vi "Send UNREGISTER.vi"(8 "error in (no error)":errorcluster, 9 "Unregister Request":T1, 10 "Message loop data (in)":T2, 11 "WAMP Client in":refnum<class "WAMP Client.lvclass">) -> (0 "error out":errorcluster, 2 "Message loop data (out)":T2, 3 "WAMP Client out":refnum<class "WAMP Client.lvclass">)   [LabVIEW 2021, in "wamplv.lvlib" / "WAMP Client.lvclass"]
uses:
  WAMP Client.lvclass
  TypeDef/Message Loop Shift Reg Data.ctl
  TypeDef/REGISTER Request Data.ctl
  API/TypeDefs/INVOCATION payload.ctl
  TypeDef/Success or error.ctl
  API/TypeDefs/Combined error.ctl
  API/TypeDefs/WAMP error.ctl
  TypeDef/Publish Requests Map.ctl
  TypeDef/PUBLISH Request Data.ctl
  TypeDef/PUBLISH result.ctl
  TypeDef/Endpoint Data.ctl
  TypeDef/CALL Request Map.ctl
  TypeDef/CALL Request Data.ctl
  API/TypeDefs/RESULT payload.ctl
  TypeDef/SUBSCRIBE Requests Map.ctl
  TypeDef/SUBSCRIBE Request Data.ctl
  TypeDef/Subscribe Result.ctl
  TypeDef/EVENT payload.ctl
  TypeDef/Subscriptions Map.ctl
  TypeDef/Subscription Details.ctl
  TypeDef/Unsubscribe Requests Map.ctl
  TypeDef/UNSUBSCRIBE Request Data.ctl
  TypeDef/UNSUBSCRIBE Result.ctl
  TypeDef/Unregister requests map.ctl
  TypeDef/Unregister request.ctl
  TypeDef/WAMP Message Codes.ctl
  WAMP Client.lvclass/WAMP Client.ctl
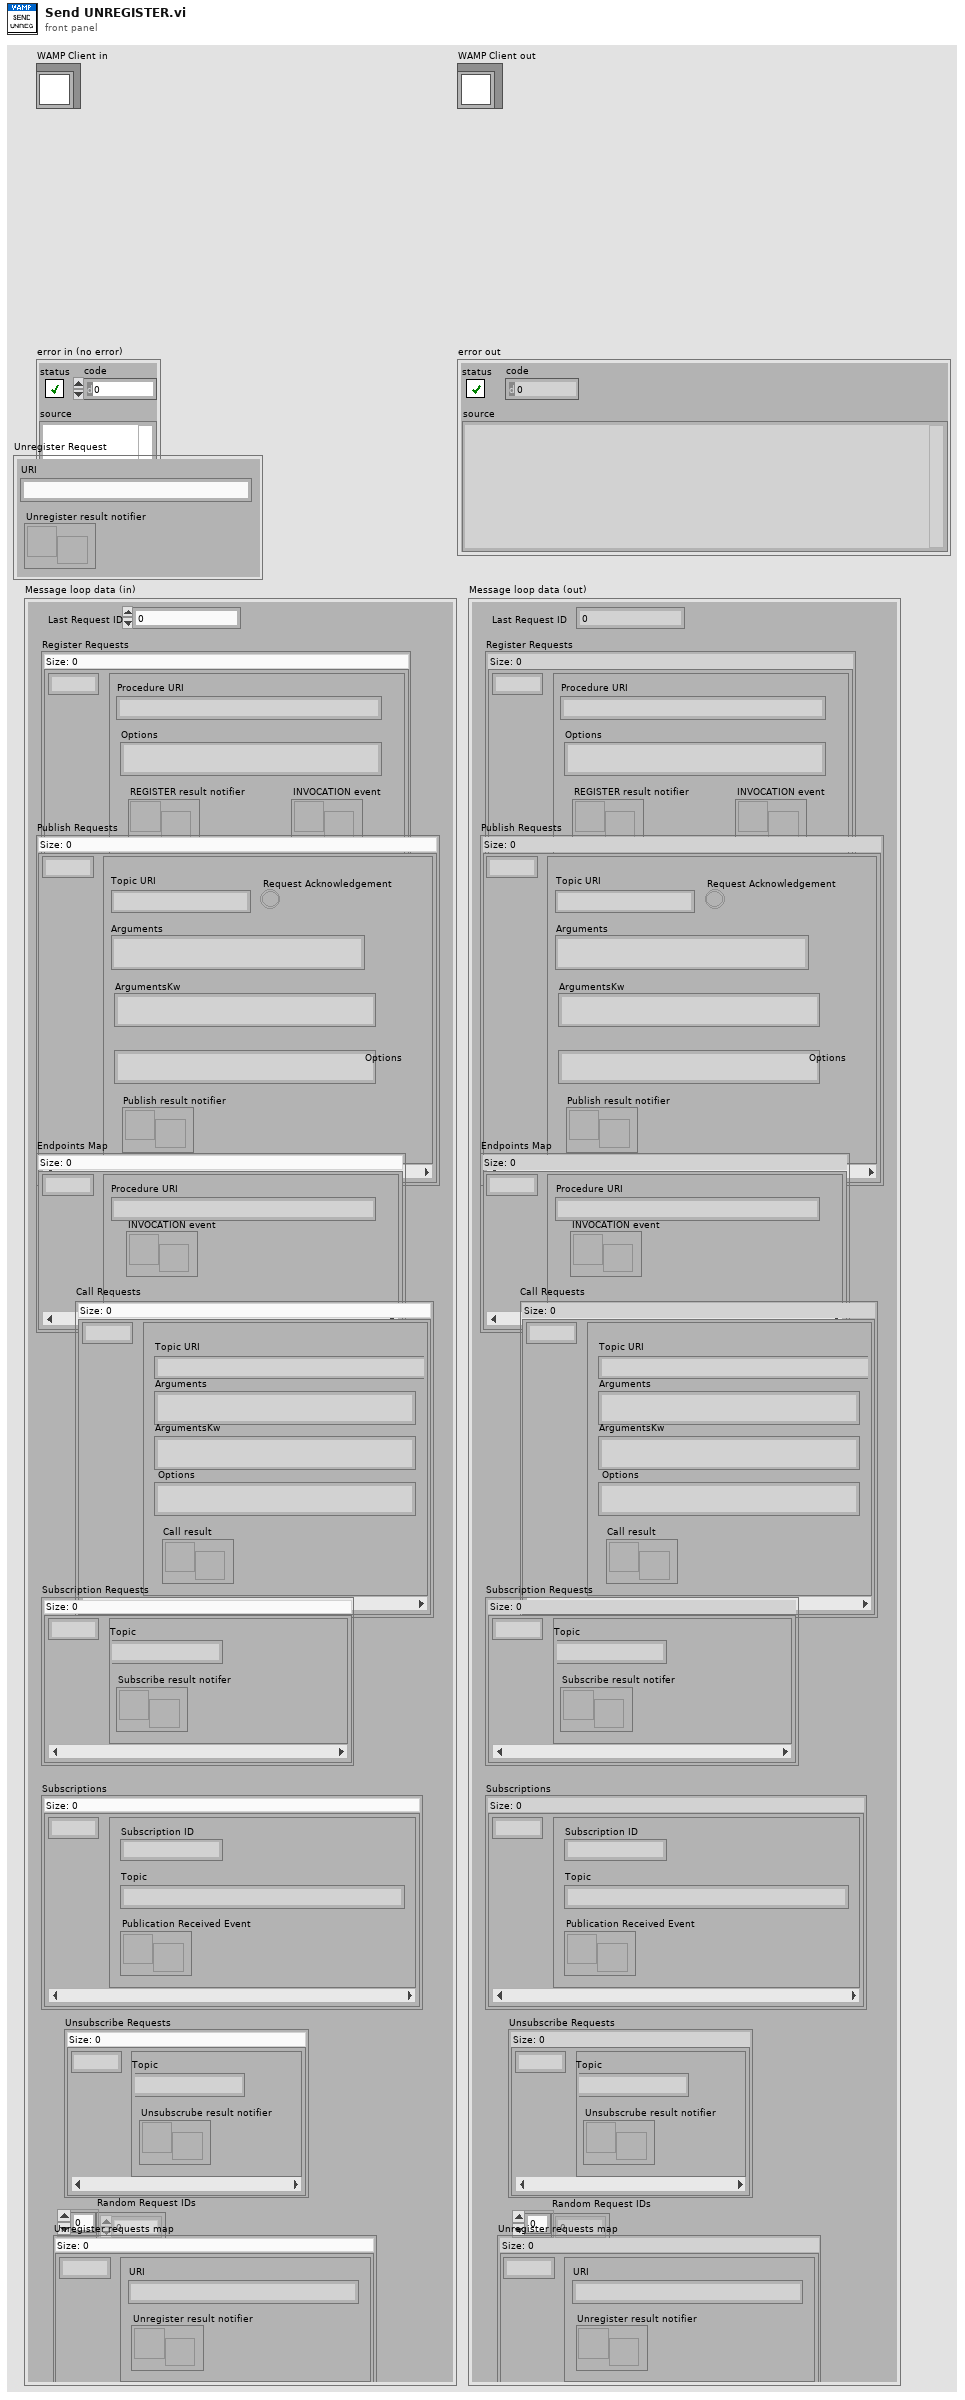
[diagram p1: front panel]
types:
  T1 = typedef "wamplv.lvlib/WAMP Client.lvclass/Unregister request.ctl" = cluster{"URI":string, "Unregister result notifier":refnum<notifier>}
  T2 = typedef "wamplv.lvlib/WAMP Client.lvclass/Message Loop Shift Reg Data.ctl" = cluster{"Last Request ID":u64, "Register Requests":map{u64, T3}, "Publish Requests":T4, "Endpoints Map":map{u64, T6}, "Call Requests":T7, "Subscription Requests":T9, "Subscriptions":T11, "Unsubscribe Requests":T13, "Random Request IDs":u64[], "Unregister requests map":T15}
  T3 = typedef "wamplv.lvlib/WAMP Client.lvclass/REGISTER Request Data.ctl" = cluster{"Procedure URI":string, "Options":string, "INVOCATION event":refnum<user-event>, "REGISTER result notifier":refnum<notifier>}
  T4 = typedef "wamplv.lvlib/WAMP Client.lvclass/Publish Requests Map.ctl" = map{u64, T5}
  T5 = typedef "wamplv.lvlib/WAMP Client.lvclass/PUBLISH Request Data.ctl" = cluster{"Topic URI":string, "Arguments":string, "ArgumentsKw":string, "Request Acknowledgement":bool, "Options":string, "Publish result notifier":refnum<notifier>}
  T6 = typedef "wamplv.lvlib/WAMP Client.lvclass/Endpoint Data.ctl" = cluster{"Procedure URI":string, "INVOCATION event":refnum<user-event>}
  T7 = typedef "wamplv.lvlib/WAMP Client.lvclass/CALL Request Map.ctl" = map{u64, T8}
  T8 = typedef "wamplv.lvlib/WAMP Client.lvclass/CALL Request Data.ctl" = cluster{"Topic URI":string, "Arguments":string, "ArgumentsKw":string, "Options":string, "Call result":refnum<notifier>}
  T9 = typedef "wamplv.lvlib/WAMP Client.lvclass/SUBSCRIBE Requests Map.ctl" = map{u64, T10}
  T10 = typedef "wamplv.lvlib/WAMP Client.lvclass/SUBSCRIBE Request Data.ctl" = cluster{"Topic":string, "Subscribe result notifer":refnum<notifier>}
  T11 = typedef "wamplv.lvlib/WAMP Client.lvclass/Subscriptions Map.ctl" = map{u64, T12}
  T12 = typedef "wamplv.lvlib/WAMP Client.lvclass/Subscription Details.ctl" = cluster{"Subscription ID":u64, "Topic":string, "Publication Received Event":refnum<user-event>}
  T13 = typedef "wamplv.lvlib/WAMP Client.lvclass/Unsubscribe Requests Map.ctl" = map{u64, T14}
  T14 = typedef "wamplv.lvlib/WAMP Client.lvclass/UNSUBSCRIBE Request Data.ctl" = cluster{"Topic":string, "Unsubscrube result notifier":refnum<notifier>}
  T15 = typedef "wamplv.lvlib/WAMP Client.lvclass/Unregister requests map.ctl" = map{u64, T1}
  T16 = typedef "wamplv.lvlib/WAMP Client.lvclass/Success or error.ctl" = cluster{"Success?":bool, "URI":string, "Combined Error":T17}
  T17 = typedef "wamplv.lvlib/WAMP Client.lvclass/Combined error.ctl" = cluster{"Error?":bool, "WAMP Error":T18, "Error":errorcluster}
  T18 = typedef "wamplv.lvlib/WAMP Client.lvclass/WAMP error.ctl" = cluster{"Details":string, "ArgumentKw Payload":string, "Error?":bool, "Error URI":string, "Arguments Payload":string}
  T19 = typedef "wamplv.lvlib/WAMP Client.lvclass/WAMP Message Codes.ctl" = u16
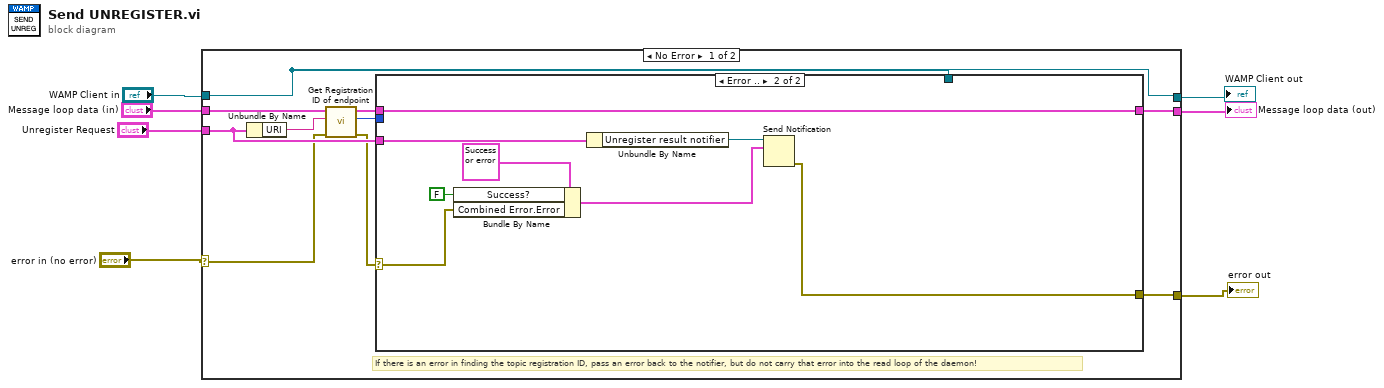
[diagram p0: block diagram]
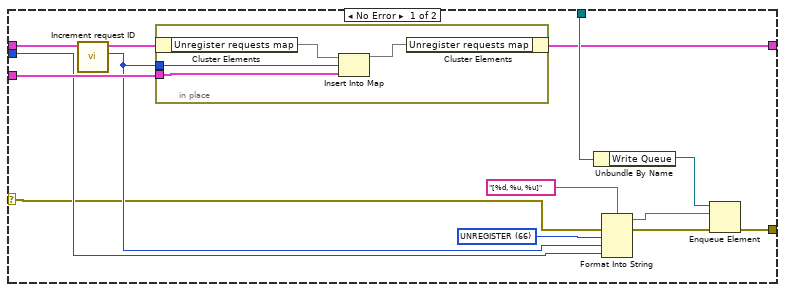
[diagram p2: hidden frame]
diagram:
  n1 = case shown="No Error" "error in (no error)" {
    selector: "error in (no error)" -> [w11 w46]
    tunnel: [w16 w46] -> w6
    tunnel: [w17 w45] -> w4
    tunnel: "WAMP Client in" -> [w17 w45]
    tunnel: "Unregister Request" -> [w15 _]
    tunnel: "Message loop data (in)" -> [w14 w44]
    tunnel: [w8 w44] -> w2
    frame No Error {
      # "If there is an error in finding the topic registration ID, pass an error back to the notifier, but do not carry that error into the read loop of the daemon!"
      n2 = Unbundle By Name(w15) -> ("URI"=w12:string)
      n3 = call "Get Registration ID of endpoint.vi"("error in"=w11, "Endpoint URI"=w12, "Message loop data (in)"=w14) -> ("error out"=w9:errorcluster, "Registrtion ID"=w10:u64, "Message loop data (out)"=w13:T2)  [unwired: 6 in]
      n4 = case shown="Error .." w9 {
        selector: w9 -> [w20 w39]
        tunnel: w17 -> [w27 _]
        tunnel: [w26 w37] -> w16
        tunnel: w15 -> [w24 w43]
        tunnel: w13 -> [w22 w42]
        tunnel: w10 -> [w21 _]
        tunnel: [w18 w42] -> w8
        frame No Error {
          w28 = T19 66 items=["HELLO"=1, "WELCOME"=2, "ABORT"=3, "GOODBYE"=6, "ERROR"=8, "PUBLISH"=16, "PUBLISHED"=17, "SUBSCRIBE"=32, "SUBSCRIBED"=33, "UNSUBSCRIBE"=34, "UNSUBSCRIBED"=35, "EVENT"=36, "CALL"=48, "RESULT"=59, "REGISTER"=64, "REGISTERED"=65, "UNREGISTER"=66, "UNREGISTERED"=67, "INVOCATION"=68, "YIELD"=70] ("Message Codes")
          n5 = call "Increment request ID.vi"("Message Loop Shift Register Data (in)"=w22) -> ("New Request ID"=w23:u64, "Message Loop Shift Register Data (out)"=w19:T2)  [unwired: 9 in]
          n6 = in-place {
            in-place-border: w24 -> [w32]
            in-place-border: w23 -> [w33]
            n7 = in-place-cluster #1(w19) -> ("Unregister requests map"=w35:T15)
            n8 = Insert Into Map(map in=w35, key=w33, value=w32) -> (map out=w34:T15)  [unwired: 2 out]
            n9 = in-place-cluster #1("Unregister requests map"=w34) -> (w18:T2)
          }
          n10 = Unbundle By Name(w27) -> ("Write Queue"=w25:refnum<queue>)
          n11 = Format Into String(format string="[%d, %u, %u]" ("element"), error in=w20, w28, w23, w21) -> (resulting string=w30:string, error out=w31:errorcluster)  [unwired: 1 in]
          n12 = Enqueue Element(queue=w25, element=w30, error in (no error)=w31) -> (error out=w26:errorcluster)  [unwired: 1 in, 2 out]
        }
        frame Error {
          n13 = Bundle By Name(cluster=T16 {"Success?"=FALSE, "URI"="", "Combined Error"={"Error?"=FALSE, "WAMP Error"={"Details"="{}", "ArgumentKw Payload"="{}", "Error?"=FALSE, "Error URI"="", "Arguments Payload"=""}, "Error"={"status"=FALSE, "code"=0, "source"=""}}} ("notification"), "Success?"=FALSE, "Combined Error.Error"=w39) -> (w38:T16)
          n14 = Unbundle By Name(w43) -> ("Unregister result notifier"=w41:refnum<notifier>)
          n15 = Send Notification(notification=w38, notifier=w41) -> (error out=w37:errorcluster)  [unwired: 1 in, 1 out]
        }
      }
    }
    frame Error {
    }
  }
  "error out" <- w6
  "WAMP Client out" <- w4
  "Message loop data (out)" <- w2
